vi "FTW-Endpoint-TCP-Reply-Worker-Start.vi"(0 "FTW-Endpoint-TCP In":refnum<class "FTW-Endpoint-TCP.lvclass">, 11 "error in":errorcluster) -> (4 "FTW-Endpoint-TCP Out":refnum<class "FTW-Endpoint-TCP.lvclass">, 15 "error out":errorcluster)   [LabVIEW 2013, in "FTW-Endpoint-TCP.lvclass"]
uses:
  FTW-Endpoint-TCP.lvclass
  FTW-Endpoint-TCP-Reply-Worker.vi
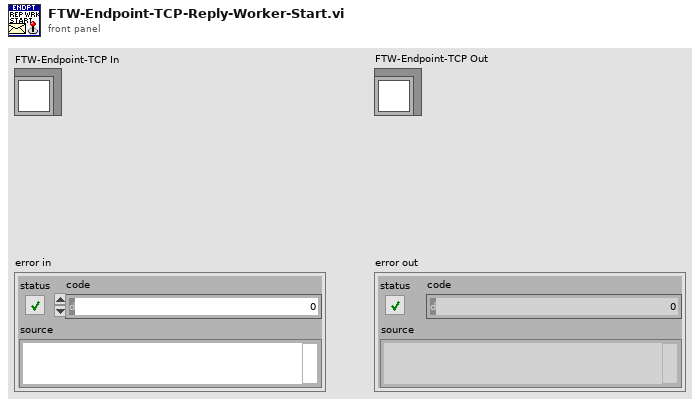
[diagram p1: front panel]
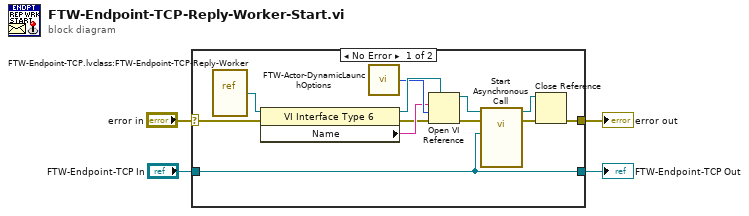
[diagram p0: block diagram]
diagram:
  n1 = case shown="No Error" "error in" {
    selector: "error in" -> [w15 w17]
    tunnel: [w16 w17] -> w1
    tunnel: "FTW-Endpoint-TCP In" -> [w5 w18]
    tunnel: [w5 w18] -> w3
    frame No Error {
      n2 = vi-ref "FTW-Endpoint-TCP.lvclass:FTW-Endpoint-TCP-Reply-Worker.vi"() -> (w6:refnum<vi>)
      n3 = property class="VI Interface Type 6"(reference=w6, error in=w15) -> (reference out=w10:refnum<vi>, error out=w7:errorcluster, "Name"=w8:string)
      n4 = call "FTW-Actor-DynamicLaunchOptions.vi"() -> ("Open VI Ref Options"=w9:i32)
      n5 = Open VI Reference(type specifier VI Refnum (for type only)=w10, vi path=w8, options=w9, error in (no error)=w7) -> (vi reference=w12:refnum<vi>, error out=w14:errorcluster)  [unwired: 2 in]
      n6 = call-by-ref "Start Asynchronous Call"(reference=w12, error in=w14, "TCP Endpoint"=w5) -> (reference out=w13:refnum<vi>, error out=w11:errorcluster)  [unwired: 15 in]
      n7 = Close Reference(reference=w13, error in (no error)=w11) -> (error out=w16:errorcluster)
    }
    frame Error {
    }
  }
  "FTW-Endpoint-TCP Out" <- w3
  "error out" <- w1
